vi "mqttCmdPingResponse.vi"(11 "error in (no error)":errorcluster) -> (15 "error out":errorcluster)   [LabVIEW 2017]
uses:
  mqttTypedef/mqttMessageType.ctl
  mqttTypedef/mqttQOSlevel.ctl
  mqttCmd.lvclass
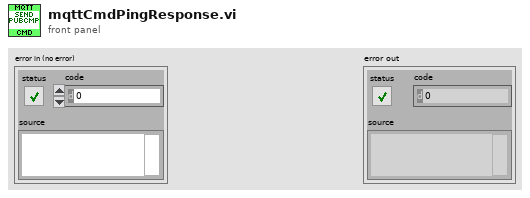
[diagram p1: front panel]
types:
  T1 = typedef "mqttQOSlevel.ctl" = enum8{"At most once", "At least once", "Exactly once", "Reserved"}
  T2 = typedef "mqttMessageType.ctl" = enum32{"Reserved", "CONNECT", "CONNACK", "PUBLISH", "PUBACK", "PUBREC", "PUBREL", "PUBCOMP", "SUBSCRIBE", "SUBACK", "UNSUBSCRIBE", "UNSUBACK", "PINGREQ", "PINGRESP", "DISCONNECT", "Reserved2"}
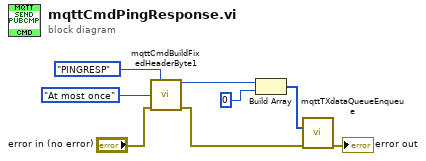
[diagram p0: block diagram]
diagram:
  n1 = call "mqttCmdBuildFixedHeaderByte1.vi"("MessageType"=mqttMessageType."PINGRESP", "QoS (At most once)"=mqttQOSlevel."At most once", "error in (no error)"="error in (no error)") -> ("byte1"=w2:u8, "error out"=w5:errorcluster)  [unwired: 11 in]
  n2 = Build Array(w2, u8 0 ("byte1")) -> (w3:u8[])
  n3 = call "mqttTXdataQueueEnqueue.vi"("data in"=w3, "error in (no error)"=w5) -> ("error out"=→"error out":errorcluster)  [unwired: 13 in]
